vi "init.vi"(8 "error in":errorcluster, 10 "TBM module configuration in":refnum<class "TBM module configuration.lvclass">, 11 "fixed channel runtime in":refnum<class "fixed channel runtime.lvclass">) -> (0 "error out":errorcluster, 1 "data allocations":T1, 2 "execution settings":T4, 3 "fixed channel runtime out":refnum<class "fixed channel runtime.lvclass">)   [LabVIEW 2013, in "fixed channel runtime.lvclass"]
doc: "Provides an interface for initializing a module at runtime. While this interface performs no operations, a child should provide an override which may open any necessary references or sessions, allocate necessary memory, and perform any final configuration validataion before providing the full configuration <b>execution data</b> to the calling process."
uses:
  fixed channel runtime.lvclass
  <vilib>/NI/Tag Bus Module Framework/module configuration/TBM module configuration.lvclass
  <vilib>/NI/Tag Bus Module Framework/runtime/execution settings.ctl
  <vilib>/NI/Tag Bus Module Framework/channel/data tables.ctl
  <vilib>/NI/Tag Bus/dictionary/data dictionary.lvclass
  <vilib>/NI/Tag Bus/dictionary table pair.ctl
  <vilib>/NI/Tag Bus/table/data table.ctl
  configuration/fixed channel configuration.lvclass
  configuration/fixed channel configuration.lvclass/fixed channel configuration.ctl
  <vilib>/NI/Tag Bus Module Framework/channel/TBM channel.lvclass
  <vilib>/NI/Tag Bus Module Framework/runtime/TBM module execution interface.lvclass
  <vilib>/NI/Tag Bus/tag bus.lvlib
  <vilib>/NI/Tag Bus/table/data table.lvlib
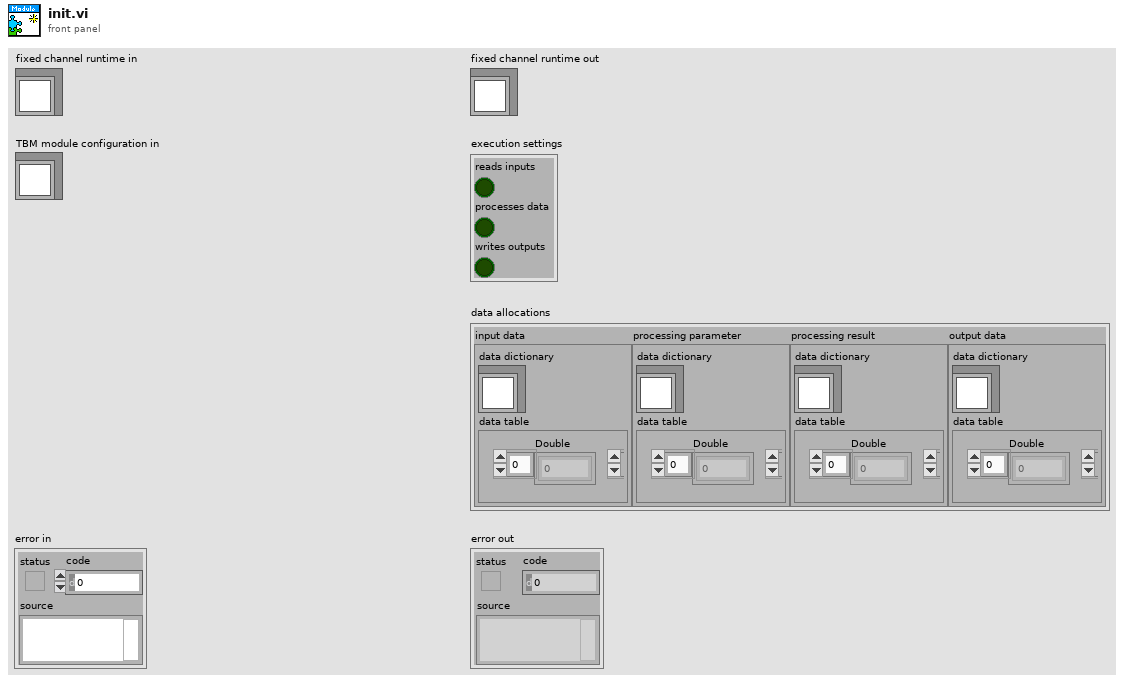
[diagram p1: front panel]
types:
  T1 = typedef "TBM channel.lvclass/data tables.ctl" = cluster{"input data":T2, "processing parameter":T2, "processing result":T2, "output data":T2}
  T2 = typedef "tag bus.lvlib/dictionary table pair.ctl" = cluster{"data dictionary":refnum<class "data dictionary.lvclass">, "data table":T3}
  T3 = typedef "tag bus.lvlib/data table.lvlib/data table.ctl" = cluster{"Double":dbl[], "Single":sgl[], "I64":i64[], "I32":i32[], "I16":i16[], "I8":i8[], "U64":u64[], "U32":u32[], "U16":u16[], "U8":u8[], "Boolean":bool[], "String":string[], "Array of Double":cluster{"DBL Array":dbl[]}[], "Array of Single":cluster{"SGL Array":sgl[]}[], "Array of I64":cluster{"I64 Array":i64[]}[], "Array of I32":cluster{"I32 Array":i32[]}[], "Array of I16":cluster{"I16 Array":i16[]}[], "Array of I8":cluster{"I8 Array":i8[]}[], "Array of U64":cluster{"U64 Array":u64[]}[], "Array of U32":cluster{"U32 Array":u32[]}[], "Array of U16":cluster{"U16 Array":u16[]}[], "Array of U8":cluster{"U8 Array":u8[]}[], "Array of Boolean":cluster{"Boolean Array":bool[]}[], "Array of String":cluster{"String Array":string[]}[]}
  T4 = typedef "TBM module execution interface.lvclass/execution settings.ctl" = cluster{"reads inputs":bool, "processes data":bool, "writes outputs":bool}
  T5 = typedef "fixed channel runtime.lvclass/Channel Run Time Mapping Info.ctl" = cluster{"Channel Indicies":i32[], "Channel Names":string[]}
  T6 = typedef "fixed channel configuration.lvclass/index type definitions.ctl" = cluster{"input indices":variant, "parameter indices":variant, "result indices":variant, "output indices":variant}
  T7 = cluster{"[0]":variant, "[1]":variant, "[2]":variant, "[3]":variant}
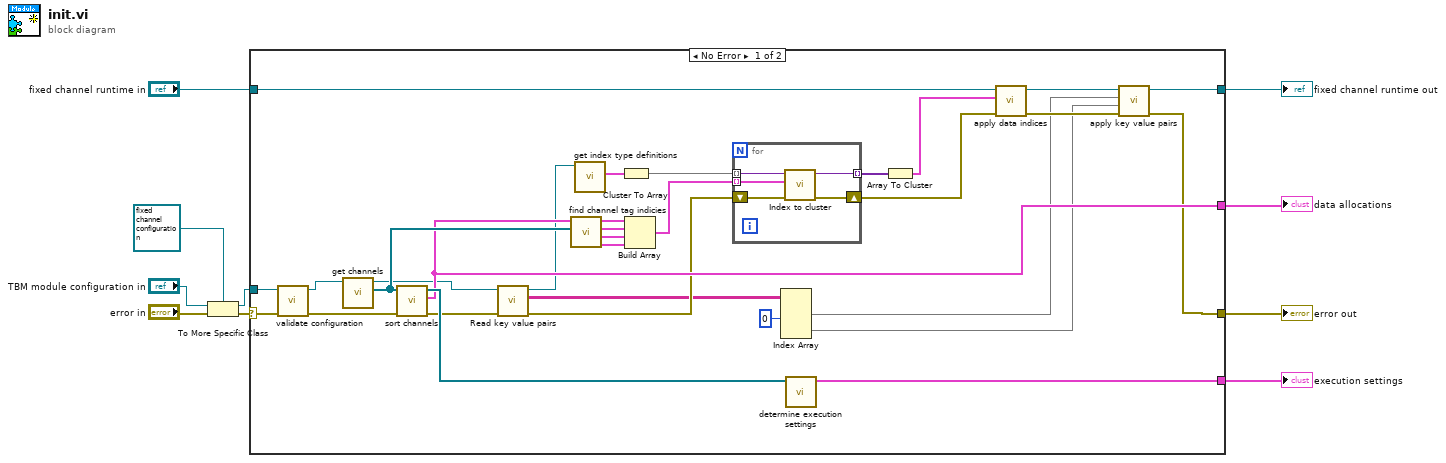
[diagram p0: block diagram]
diagram:
  n1 = To More Specific Class(target class=refnum<class "fixed channel configuration.lvclass"> refnum ("Synchronous module configuration"), reference="TBM module configuration in", error in="error in") -> (specific class reference=w1:refnum<class "fixed channel configuration.lvclass">, error out=w2:errorcluster)
  n2 = case shown="No Error" w2 {
    selector: w2 -> [w39 w47]
    tunnel: w1 -> [w38 _]
    tunnel: "fixed channel runtime in" -> [w26 w48]
    tunnel: [w19 w48] -> w8
    tunnel: [w21 w47] -> w7
    tunnel: [w34 _] -> w5
    tunnel: [w41 _] -> w6
    frame No Error {
      n3 = call-dynamic "validate configuration.vi"("error in"=w39, "fixed channel configuration in"=w38) -> ("error out"=w40:errorcluster, "fixed channel configuration out"=w37:refnum<class "fixed channel configuration.lvclass">)  [unwired: 8 in]
      n4 = call-dynamic "get channels.vi"("fixed channel configuration in"=w37) -> ("channels"=w35:refnum<class "TBM channel.lvclass">[], "fixed channel configuration out"=w16:refnum<class "fixed channel configuration.lvclass">)  [unwired: 9 in]
      n5 = call <vilib>:"sort channels.vi"("error in"=w40, "channels in"=w35) -> ("error out"=w18:errorcluster, "data allocations"=w34:T1, "channels out"=w36:refnum<class "TBM channel.lvclass">[])  [unwired: 7 in]
      n6 = call "Read key value pairs.vi"("error in"=w18, "fixed channel configuration in"=w16) -> ("error out"=w17:errorcluster, "key value pairs"=w14:string[][], "fixed channel configuration out"=w15:refnum<class "fixed channel configuration.lvclass">)  [unwired: 7 in]
      n7 = call "find channel tag indicies.vi"("channels"=w35, "data allocations"=w34) -> ("Output Indicies"=w33:T5, "Result Indicies"=w32:T5, "Parameter Indicies"=w31:T5, "Input Indicies"=w30:T5)  [unwired: 6 in]
      n8 = call-dynamic "get index type definitions.vi"("fixed channel configuration in"=w15) -> ("index type defs"=w29:T6)  [unwired: 9 in, 1 out]
      n9 = Cluster To Array(cluster=w29) -> (array=w28:variant[])
      n10 = Build Array(w30, w31, w32, w33) -> (w27:T5[])
      n11 = for {
        tunnel: w28 -> [w46] mode=indexing
        tunnel: w27 -> [w45] mode=indexing
        tunnel: [w44] -> w25 mode=indexing
        shift-right: [w43] -> w22
        shift-left: w17 -> [w42]
        n12 = call "Index to cluster.vi"("error in"=w42, "Input Mapping Info"=w45, "Variant in"=w46) -> ("error out"=w43:errorcluster, "Variant out"=w44:variant)  [unwired: 7 in]
      }
      n13 = Index Array(array=w14, index (col) #1=0 ("disabled index (col)")) -> (element #1=w12:string[], element #2=w11:string[])  [unwired: 3 in]
      n14 = call <vilib>:"determine execution settings.vi"("channels"=w36) -> ("execution settings"=w41:T4)  [unwired: 10 in]
      n15 = Array To Cluster(array=w25) -> (cluster=w24:T7)
      n16 = call-dynamic "apply data indices.vi"("error in"=w22, "index type defs"=w24, "fixed channel runtime in"=w26) -> ("error out"=w23:errorcluster, "fixed channel runtime out"=w20:refnum<class "fixed channel runtime.lvclass">)  [unwired: 7 in]
      n17 = call-dynamic "apply key value pairs.vi"("error in"=w23, "values"=w11, "keys"=w12, "fixed channel runtime in"=w20) -> ("error out"=w21:errorcluster, "fixed channel runtime out"=w19:refnum<class "fixed channel runtime.lvclass">)  [unwired: 6 in]
    }
    frame Error {
    }
  }
  "error out" <- w7
  "fixed channel runtime out" <- w8
  "execution settings" <- w6
  "data allocations" <- w5
